vi "Leddar2LabVIEW.vi"() -> ()   [LabVIEW 2012]
panel:
  in  "Stop Run":bool
  in  "btnStop":bool
  in  "btnStart":bool
  in  "Connection Mode":enum32{"INIT_FILE", "INIT_LIVE"}(radio)
  in  "USB Device Name":string="AC12345"
  in  "Path to Record":path=path "D:/R&D-2013-06-19-14-07-16-824.ltl"
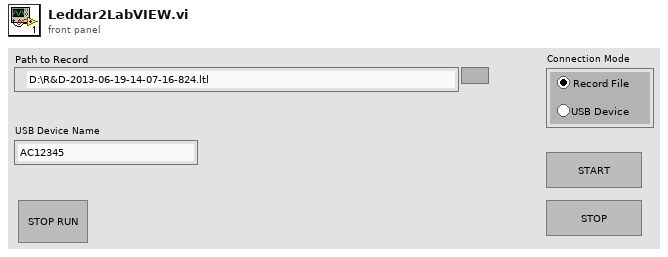
[diagram p1: front panel]
types:
  T1 = enum8{"Enabled", "Disabled", "Disabled and Grayed Out"}
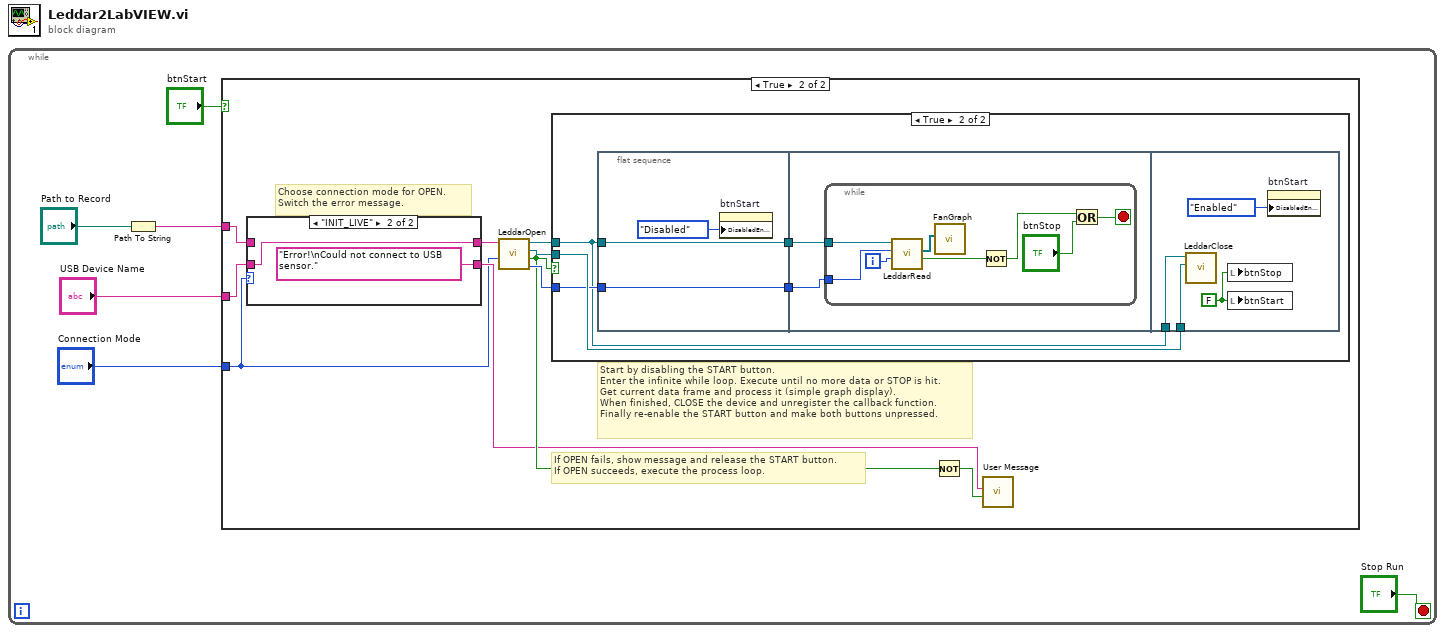
[diagram p0: block diagram]
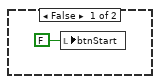
[diagram p3: hidden frame]
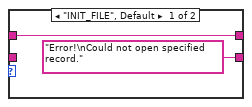
[diagram p4: hidden frame]
diagram:
  n1 = while {
    stop <- "Stop Run" stop-if-true
    n2 = Path To String(path="Path to Record") -> (string=w3:string)
    n3 = case shown="True" "btnStart" {
      tunnel: "Connection Mode" -> [_ w7]
      tunnel: w3 -> [_ w16]
      tunnel: "USB Device Name" -> [_ w15]
      frame False {
      }
      frame True {
        # "Start by disabling the START button.\nEnter the infinite while loop. Execute until no more data or STOP is hit.\nGet current data frame and process it (simple graph display).\nWhen finished, CLOSE the device and unregister the callback function.\nFinally re-enable the START button and make both buttons unpressed."
        # "If OPEN fails, show message and release the START button.\nIf OPEN succeeds, execute the process loop."
        # "Choose connection mode for OPEN.\nSwitch the error message."
        n4 = case shown="\"INIT_LIVE\"" w7 {
          tunnel: w16 -> [w41 _]
          tunnel: w15 -> [_ w43]
          tunnel: [w41 w43] -> w12
          tunnel: ["Error!\nCould not open specified record." "Error!\nCould not connect to USB sensor."] -> w11
          frame "INIT_FILE", Default {
          }
          frame "INIT_LIVE" {
          }
        }
        n5 = call "LeddarOpen.vi"("Connection Mode"=w7, "File path, USB name"=w12) -> ("Connection Mode Out"=w14:enum32{"INIT_FILE", "INIT_LIVE"}, "Success"=w13:bool, "Event Callback"=w9:refnum<k27>, "DeviceControl"=w8:refnum<k24>)  [unwired: 6 in]
        n6 = case shown="True" w13 {
          tunnel: w14 -> [_ w21]
          tunnel: w9 -> [_ w22]
          tunnel: w8 -> [_ w20]
          frame False {
            n7 = local write "btnStart"(FALSE) -> ()
          }
          frame True {
            n8 = flat-sequence {
              tunnel: w20 -> [w24]
              tunnel: w21 -> [w25]
              tunnel: [w25] -> w19
              tunnel: [w24] -> w18
              tunnel: w19 -> [w27]
              tunnel: w18 -> [w26]
              tunnel: w20 -> [w36]
              tunnel: w22 -> [w37]
              frame #0 {
                n9 = property on="btnStart" class="Bool (strict)"("DisabledEnum"=T1."Disabled" ("Disabled")) -> ()  [unwired: 2 in, 2 out]
              }
              frame #1 {
                n10 = while {
                  tunnel: w27 -> [w31]
                  tunnel: w26 -> [w30]
                  i -> [w32]
                  stop <- w33 stop-if-true
                  n11 = call "LeddarRead.vi"("Frame Index"=w32, "Connection Mode"=w31, "DeviceControl"=w30) -> ("New Status"=w29:bool, "Detections Array"=w28:refnum<k24>[])  [unwired: 6 in, 1 out]
                  n12 = call "FanGraph.vi"("Detections"=w28) -> ()  [unwired: 9 in, 1 out]
                  n13 = Not(x=w29) -> (.not. x?=w34:bool)
                  n14 = Or(x=w34, y="btnStop") -> (x .or. y?=w33:bool)
                }
              }
              frame #2 {
                w38 = FALSE
                n15 = call "LeddarClose.vi"("Event Callback"=w37, "DeviceControl"=w36) -> ()  [unwired: 10 in]
                n16 = local write "btnStop"(w38) -> ()
                n17 = local write "btnStart"(w38) -> ()
                n18 = property on="btnStart" class="Bool (strict)"("DisabledEnum"=T1."Enabled" ("Disabled")) -> ()  [unwired: 2 in, 2 out]
              }
            }
          }
        }
        n19 = Not(x=w13) -> (.not. x?=w10:bool)
        n20 = call "User Message"("Enable"=w10, "Message"=w11) -> ()  [unwired: 8 in, 2 out]
      }
    }
  }
